vi "GamePiecePose.vi"(0 "GamePiece Valid [t-?]":bool, 1 "Robot Heading (deg)":dbl, 2 "Odometry Timestamp (ms)":u32, 3 "GamePiece Timestamp (ms)":u32, 5 "GamePiece Type [t-?]":enum16{"None", "Cube", "Cone"}(ring), 7 "Y (in) [t0]":dbl, 9 "X (in) [t0]":dbl, 12 "GamePiece Ty (deg) [t-?]":dbl, 13 "GamePiece Tx (deg) [t-?]":dbl) -> (4 "GamePiece Y (in) [t-?]":dbl, 6 "GamePiece X (in) [t-?]":dbl, 8 "GamePiece Valid [t-?]":bool, 10 "GamePiece Range (in) [t-?":dbl)   [LabVIEW 2020]
doc: "Calculates the detected game piece pose relative to the robot using data from the LimeLight camera. Also performs additional validation checks to determine if the game piece vision data should be trusted."
uses:
  54abcb88-3220-419e-9bec-4c3c6f5e2905.vi
  76103391-ba62-4dc0-bcc0-26de5557a5b7.vi
  e823d307-d35b-45d7-a729-51121ade1bdb.vi
  4f3d002f-ad2c-48f1-81b6-0e59c3cd0741.vi
  GlobalPoseAndTargeting.vi
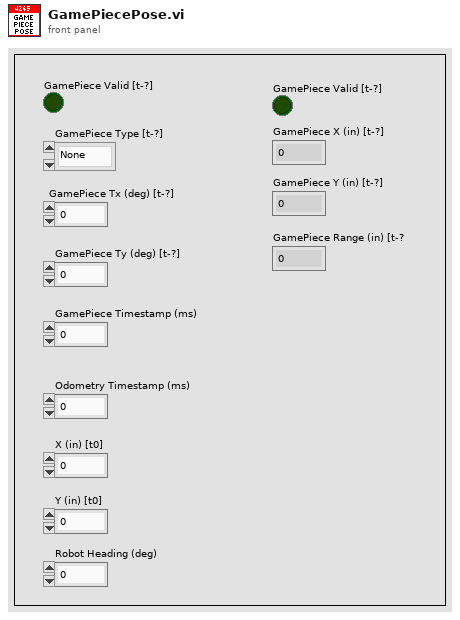
[diagram p1: front panel]
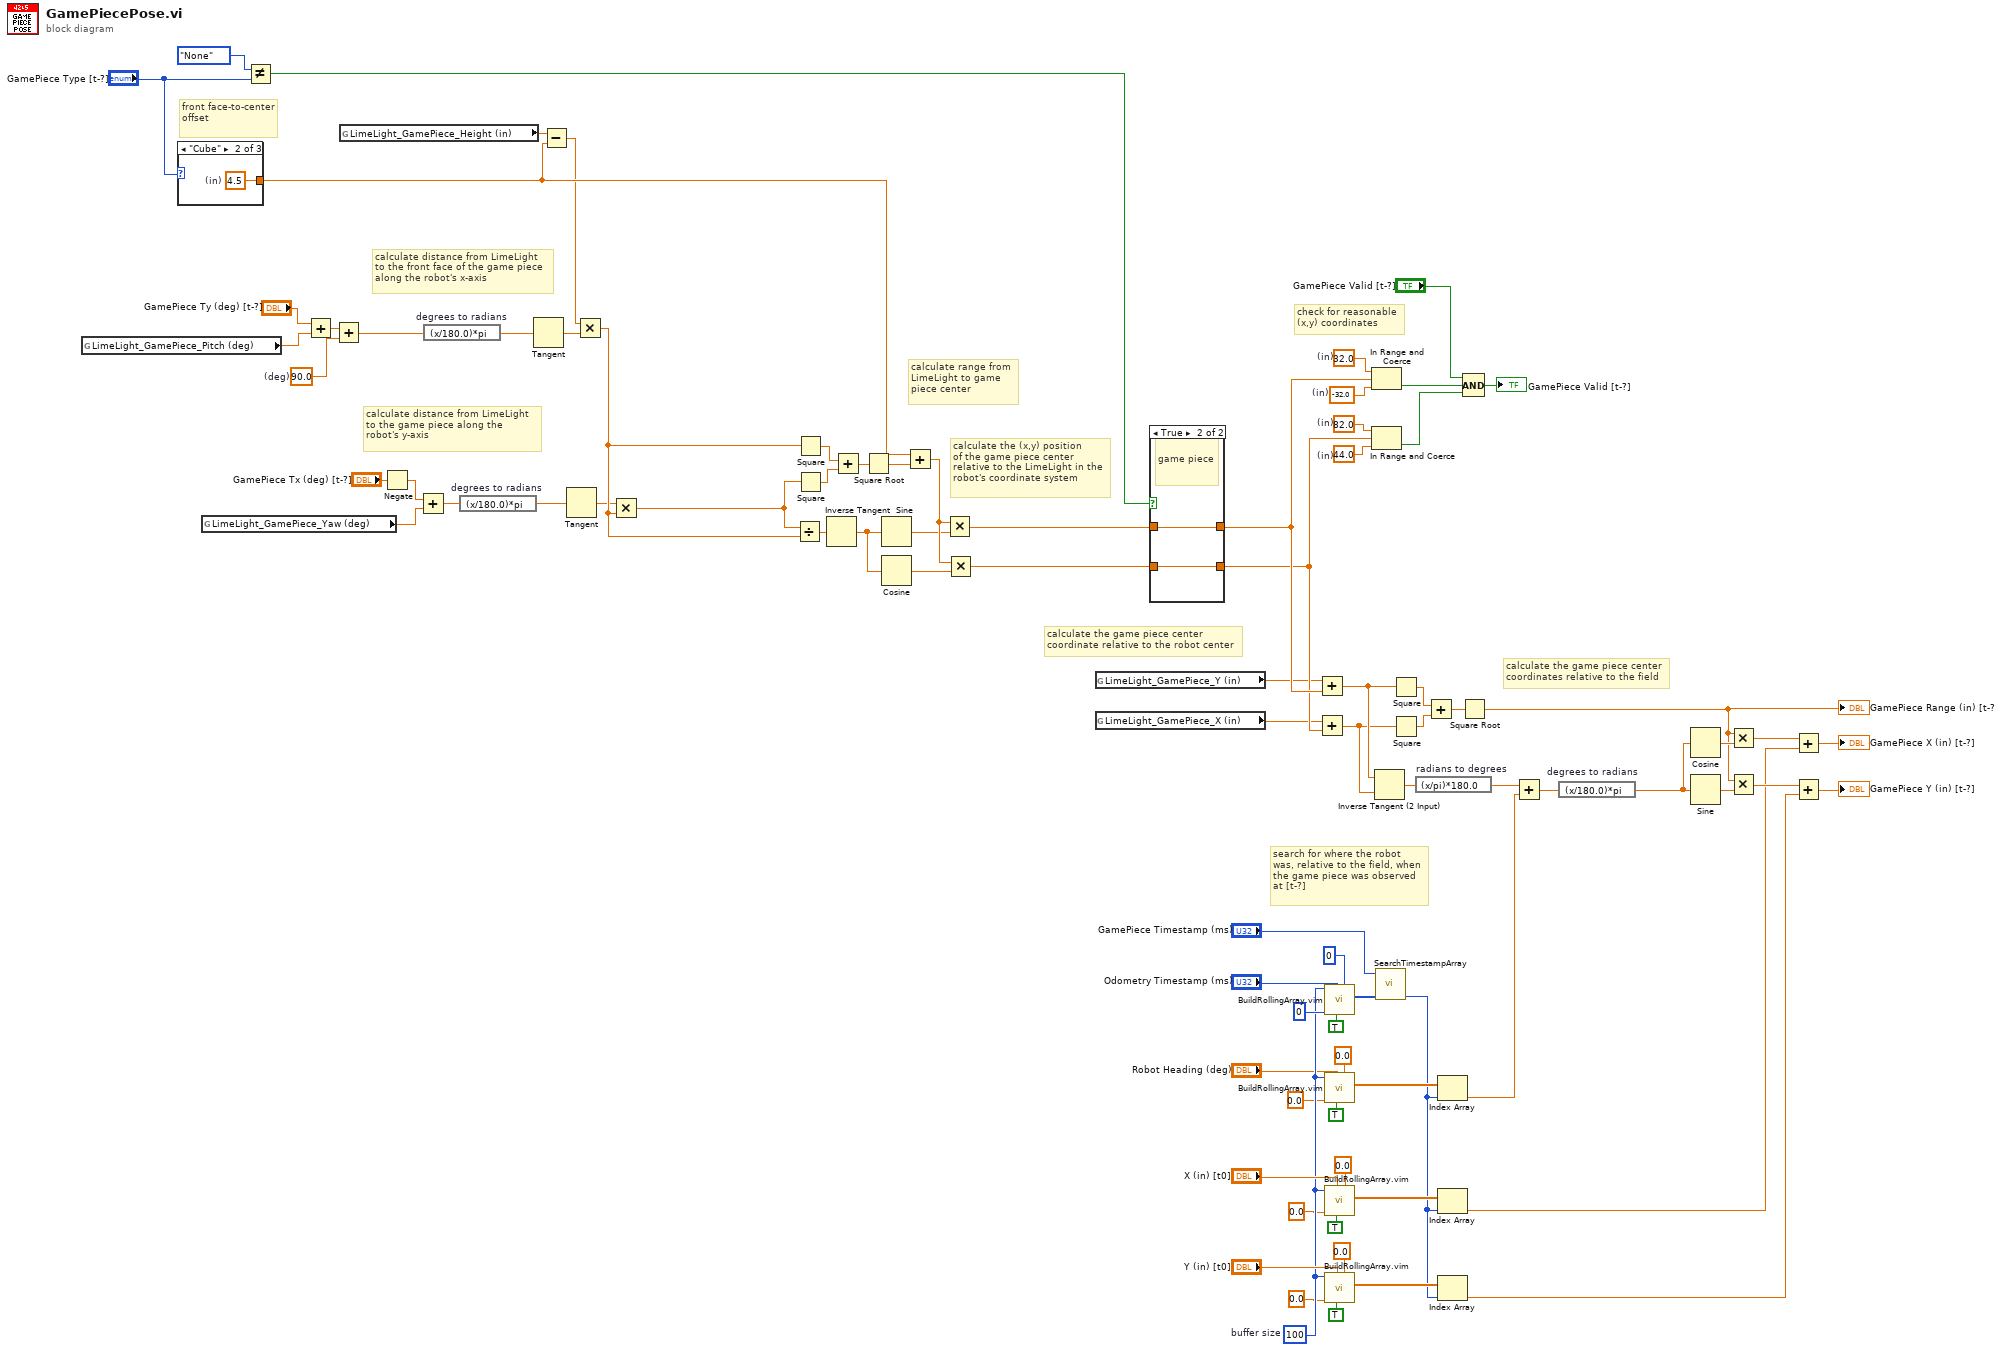
[diagram p0: block diagram]
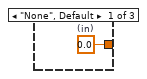
[diagram p2: hidden frame]
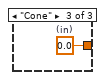
[diagram p3: hidden frame]
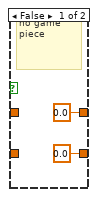
[diagram p4: hidden frame]
diagram:
  w34 = 100  # buffer size
  w59 = 44.0  # (in)
  w60 = 82.0  # (in)
  w61 = -32.0  # (in)
  w62 = 32.0  # (in)
  w73 = 90.0  # (deg)
  # "search for where the robot\nwas, relative to the field, when\nthe game piece was observed\nat [t-?]"
  # "calculate the game piece center\ncoordinates relative to the field"
  # "check for reasonable\n(x,y) coordinates"
  # "calculate the game piece center\ncoordinate relative to the robot center"
  # "calculate the (x,y) position\nof the game piece center \nrelative to the LimeLight in the\nrobot's coordinate system"
  # "calculate range from\nLimeLight to game\npiece center"
  # "calculate distance from LimeLight\nto the game piece along the\nrobot's y-axis"
  # "calculate distance from LimeLight\nto the front face of the game piece\nalong the robot's x-axis"
  # "front face-to-center offset"
  n1 = global read "GlobalPoseAndTargeting.vi" "LimeLight_GamePiece_Pitch (deg)"() -> (w19:dbl)
  n2 = case shown="\"Cube\"" "GamePiece Type [t-?]" {
    tunnel: [w87 w88 w89] -> w3
    frame "None", Default {
      w87 = 0.0  # (in)
    }
    frame "Cube" {
      w88 = 4.5  # (in)
    }
    frame "Cone" {
      w89 = 0.0  # (in)
    }
  }
  n3 = global read "GlobalPoseAndTargeting.vi" "LimeLight_GamePiece_Yaw (deg)"() -> (w68:dbl)
  n4 = Not Equal?(x=enum16{"None", "Cube", "Cone"}."None" ("y"), y="GamePiece Type [t-?]") -> (x != y?=w70:bool)
  n5 = Add(x="GamePiece Ty (deg) [t-?]", y=w19) -> (x+y=w23:dbl)
  n6 = Add(x=w23, y=w73) -> (x+y=w72:dbl)
  n7 = global read "GlobalPoseAndTargeting.vi" "LimeLight_GamePiece_Height (in)"() -> (w4:dbl)
  n8 = Negate(x="GamePiece Tx (deg) [t-?]") -> (-x=w56:dbl)
  n9 = Add(x=w56, y=w68) -> (x+y=w74:dbl)
  n10 = expression code="(x/180.0)*pi" "degrees to radians"(w72) -> (w71:dbl)
  n11 = expression code="(x/180.0)*pi" "degrees to radians"(w74) -> (w75:dbl)
  n12 = Tangent(1:w71) -> (0:w2:dbl)
  n13 = Subtract(x=w4, y=w3) -> (x-y=w1:dbl)
  n14 = Tangent(1:w75) -> (0:w76:dbl)
  n15 = Multiply(x=w1, y=w2) -> (x*y=w82:dbl)
  n16 = Multiply(x=w76, y=w82) -> (x*y=w83:dbl)
  n17 = Divide(x=w83, y=w82) -> (x/y=w78:dbl)
  n18 = Square(x=w82) -> (x^2=w15:dbl)
  n19 = Square(x=w83) -> (x^2=w14:dbl)
  n20 = Inverse Tangent(1:w78) -> (0:w80:dbl)
  n21 = Add(x=w15, y=w14) -> (x+y=w77:dbl)
  n22 = Square Root(x=w77) -> (sqrt(x)=w13:dbl)
  n23 = Sine(x=w80) -> (sin(x)=w79:dbl)
  n24 = Cosine(x=w80) -> (cos(x)=w81:dbl)
  n25 = Add(x=w3, y=w13) -> (x+y=w84:dbl)
  n26 = Multiply(x=w84, y=w79) -> (x*y=w85:dbl)
  n27 = Multiply(x=w84, y=w81) -> (x*y=w86:dbl)
  n28 = global read "GlobalPoseAndTargeting.vi" "LimeLight_GamePiece_Y (in)"() -> (w58:dbl)
  n29 = global read "GlobalPoseAndTargeting.vi" "LimeLight_GamePiece_X (in)"() -> (w57:dbl)
  n30 = case shown="True" w70 {
    tunnel: w85 -> [_ w93]
    tunnel: [0.0 w93] -> w67
    tunnel: w86 -> [_ w92]
    tunnel: [0.0 w92] -> w66
    frame False {
      # "no game piece"
    }
    frame True {
      # "game piece"
    }
  }
  n31 = Add(x=w58, y=w67) -> (x+y=w22:dbl)
  n32 = Add(x=w57, y=w66) -> (x+y=w21:dbl)
  n33 = call "BuildRollingArray.vim"("Global Additive Update"=0, "Update?"=TRUE, "New Value"="Odometry Timestamp (ms)", "Initial Value"=0, "Number of Elements"=w34) -> ("Current Array"=w46:u32[])  [unwired: 6 in]
  n34 = call "BuildRollingArray.vim"("Global Additive Update"=0.0, "Update?"=TRUE, "New Value"="Robot Heading (deg)", "Initial Value"=0.0, "Number of Elements"=w34) -> ("Current Array"=w36:dbl[])  [unwired: 6 in]
  n35 = call "BuildRollingArray.vim"("Global Additive Update"=0.0, "Update?"=TRUE, "New Value"="X (in) [t0]", "Initial Value"=0.0, "Number of Elements"=w34) -> ("Current Array"=w45:dbl[])  [unwired: 6 in]
  n36 = call "BuildRollingArray.vim"("Global Additive Update"=0.0, "Update?"=TRUE, "New Value"="Y (in) [t0]", "Initial Value"=0.0, "Number of Elements"=w34) -> ("Current Array"=w44:dbl[])  [unwired: 6 in]
  n37 = In Range and Coerce(upper limit=w62, x=w67, lower limit=w61) -> (In Range?=w64:bool)  [unwired: 1 out]
  n38 = In Range and Coerce(upper limit=w60, x=w66, lower limit=w59) -> (In Range?=w63:bool)  [unwired: 1 out]
  n39 = Inverse Tangent (2 Input)(1:w21, 2:w22) -> (0:w17:dbl)
  n40 = call "SearchTimestampArray.vi"("Timestamp Array"=w46, "Search Timestamp"="GamePiece Timestamp (ms)") -> ("Closest Index"=w35:i32)  [unwired: 8 in, 1 out]
  n41 = Square(x=w22) -> (x^2=w50:dbl)
  n42 = Square(x=w21) -> (x^2=w51:dbl)
  n43 = expression code="(x/pi)*180.0" "radians to degrees"(w17) -> (w16:dbl)
  n44 = Add(x=w50, y=w51) -> (x+y=w52:dbl)
  n45 = Index Array(array=w36, index=w35) -> (element=w32:dbl)
  n46 = Index Array(array=w45, index=w35) -> (element=w25:dbl)
  n47 = Index Array(array=w44, index=w35) -> (element=w24:dbl)
  n48 = Square Root(x=w52) -> (sqrt(x)=w18:dbl)
  "GamePiece Range (in) [t-?" <- w18
  n49 = Compound Arithmetic op=AND("GamePiece Valid [t-?]", w64, w63) -> (→"GamePiece Valid [t-?]":bool)
  n50 = Add(x=w16, y=w32) -> (x+y=w49:dbl)
  n51 = expression code="(x/180.0)*pi" "degrees to radians"(w49) -> (w53:dbl)
  n52 = Cosine(x=w53) -> (cos(x)=w54:dbl)
  n53 = Sine(x=w53) -> (sin(x)=w55:dbl)
  n54 = Multiply(x=w18, y=w54) -> (x*y=w26:dbl)
  n55 = Multiply(x=w18, y=w55) -> (x*y=w27:dbl)
  n56 = Add(x=w26, y=w25) -> (x+y=→"GamePiece X (in) [t-?]":dbl)
  n57 = Add(x=w27, y=w24) -> (x+y=→"GamePiece Y (in) [t-?]":dbl)
